vi "Array to XY Graph.vi"(0 "2DArray":ext[][](array[numeric])) -> (2 "XY Graph object":cluster{ext[], ext[]})   [LabVIEW 2009]
doc: "Translates a 2D array into a graph object. The array has 2 columns: x-values in column 1, y-values in column 2. That is, each row of the array represents a point on the graph with appropriate x and y coordinates."
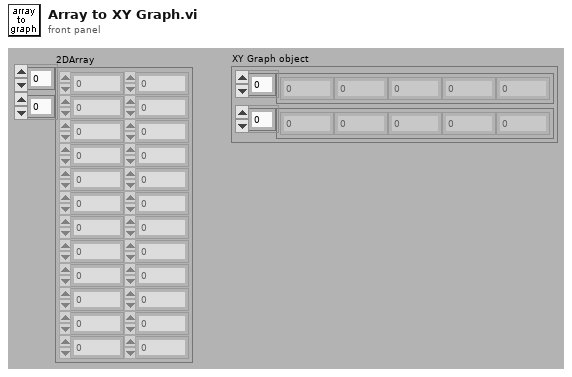
[diagram p1: front panel]
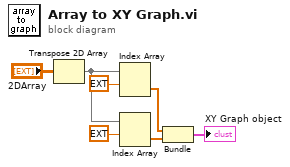
[diagram p0: block diagram]
diagram:
  n1 = Transpose 2D Array(2D array="2DArray") -> (transposed array=w4:ext[][])
  n2 = Index Array(array=w4, index (row)=ext 0.0 ("index")) -> (element=w5:ext[])  [unwired: 1 in]
  n3 = Index Array(array=w4, index (row)=ext 1.0 ("index")) -> (element=w6:ext[])  [unwired: 1 in]
  n4 = Bundle(w5, w6) -> (→"XY Graph object":cluster{ext[], ext[]})  [unwired: 1 in]
